vi "HV507 Write - Alt.vi"(8 "Error In":errorcluster, 10 "HV Data Bitmask":u64, 11 "LINX Resource":T1) -> (0 "Error Out":errorcluster, 3 "LINX Resource 2":T1)   [LabVIEW 2017]
doc: "Write 64-bit data to the 64 high voltage output channels of HV507.\n\nThis VI takes a 64 bit unigned integer as input and writes the bitwise data to HV507.\n\nArduino Microcontroller pins configured as follows:\nDIO 7 - ~BL\nDIO 8 - ~LE\nDIO 11 - DI\nDIO 13 - SCLK"
uses:
  <vilib>/MakerHub/LINX/Private/Type Defs/LINX Ref.ctl
  <vilib>/MakerHub/LINX/Private/Type Defs/Platform.ctl
  <vilib>/MakerHub/LINX/Private/Type Defs/Interface.ctl
  <vilib>/MakerHub/LINX/Private/Device/Type Defs/LINX Device Config.ctl
  <vilib>/MakerHub/LINX/Private/Device/Type Defs/TCP Config.ctl
  <vilib>/MakerHub/LINX/Private/Device/Type Defs/Channels.ctl
  <vilib>/MakerHub/LINX/Private/Type Defs/Peripherals/SPI/SPI Configuration.ctl
  <vilib>/MakerHub/LINX/Private/Type Defs/Peripherals/SPI/SPI Bit Order.ctl
  <vilib>/MakerHub/LINX/Private/Type Defs/Peripherals/SPI/SPI Mode.ctl
  <vilib>/MakerHub/LINX/Public/Peripherals/SPI/SPI CS Config.ctl
  <vilib>/MakerHub/LINX/Private/Type Defs/Peripherals/SPI/SPI CS Logic Level.ctl
  <vilib>/MakerHub/LINX/Public/Peripherals/SPI/SPI Write Read 1 Frame.vi
  <vilib>/MakerHub/LINX/Public/Peripherals/SPI/SPI Write Read N Frames.vi
  <vilib>/MakerHub/LINX/Private/Local IO/LinxSpiWriteRead.vi
  <vilib>/MakerHub/LINX/Public/Utilities/Check Channel.vi
  <vilib>/MakerHub/LINX/Private/Utilties/Generate Error.vi
  <vilib>/MakerHub/LINX/LMH-LINX.lvlib
  <vilib>/MakerHub/LINX/Private/Device/Device.lvlib
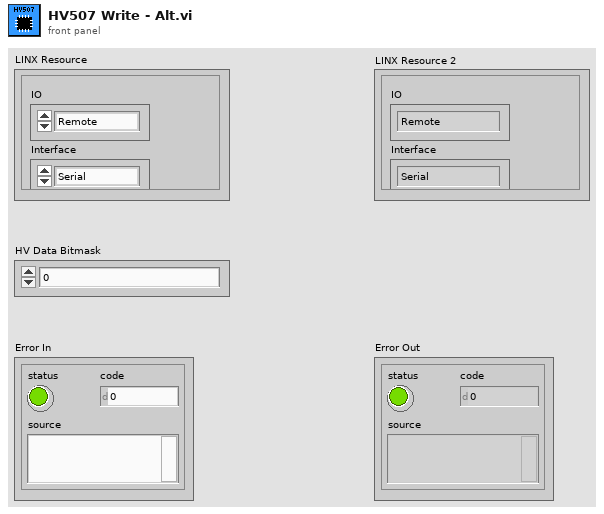
[diagram p1: front panel]
types:
  T1 = typedef "LMH-LINX.lvlib/LINX Ref.ctl" = cluster{"IO":T2, "Interface":T3, "LINX Device Config":T4}
  T2 = typedef "LMH-LINX.lvlib/Platform.ctl" = enum16{"Remote", "Local"}
  T3 = typedef "LMH-LINX.lvlib/Interface.ctl" = enum16{"Serial", "TCP"}
  T4 = typedef "LMH-LINX.lvlib/Device.lvlib/LINX Device Config.ctl" = cluster{"Interface":T3, "COM Port":refnum<visa-resource-name>, "TCP Configuration":T5, "Device Family":u8, "Device ID":u8, "Device Name":string, "TCP Ref":refnum<k5>, "Channels":T6}
  T5 = typedef "LMH-LINX.lvlib/Device.lvlib/TCP Config.ctl" = cluster{"IP Address":string, "Port":u16}
  T6 = typedef "LMH-LINX.lvlib/Channels.ctl" = cluster{"DI":u8[], "DO":u8[], "AI":u8[], "AO":u8[], "PWM":u8[], "QE":u8[], "UART":u8[], "I2C 2":u8[], "SPI":u8[], "CAN":u8[], "Servo":u8[], "AI Ref (V)":dbl, "AI Resolution (Bits)":u8, "AO Ref (V)":dbl, "AO Resolution (Bits)":u8}
  T7 = typedef "LMH-LINX.lvlib/SPI CS Config.ctl" = cluster{"CS Channel":u8, "CS Logic Level":T8}
  T8 = typedef "LMH-LINX.lvlib/SPI CS Logic Level.ctl" = enum8{"Active Low", "Active High"}
  T9 = typedef "LMH-LINX.lvlib/SPI Configuration.ctl" = cluster{"Clock Frequency":u32, "Bit Order":T10, "SPI Mode":T11}
  T10 = typedef "LMH-LINX.lvlib/SPI Bit Order.ctl" = enum8{"LSb First", "MSb First"}
  T11 = typedef "LMH-LINX.lvlib/SPI Mode.ctl" = enum8{"Mode 0", "Mode 1", "Mode 2", "Mode 3"}
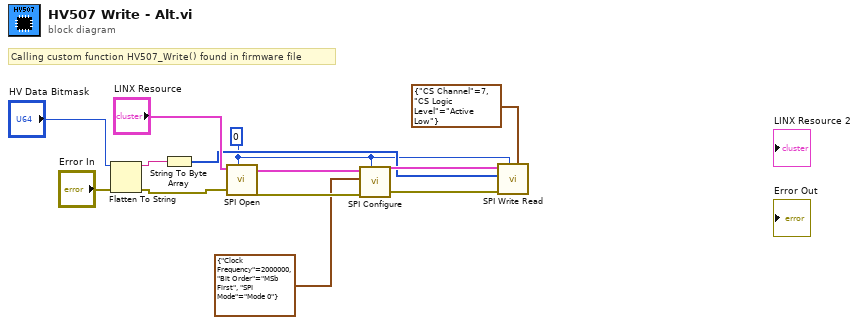
[diagram p0: block diagram]
diagram:
  w2 = u8 0 ("SPI Channel (0)")
  # "Calling custom function HV507_Write() found in firmware file"
  n1 = Flatten To String(anything="HV Data Bitmask", error in (no error)="Error In") -> (data string=w11:string, error out=w10:errorcluster)  [unwired: 2 in, 1 out]
  n2 = String To Byte Array(string=w11) -> (unsigned byte array=w3:u8[])
  n3 = call <vilib>:"SPI Open.vi"("SPI Channel (0)"=w2, "Error In"=w10, "LINX Resource"="LINX Resource") -> ("Error Out"=w8:errorcluster, "LINX Resource"=w7:T1)  [unwired: 7 in]
  n4 = call <vilib>:"SPI Configure.vi"("SPI Channel (0)"=w2, "Error In"=w8, "SPI Configuration"=T9 {"Clock Frequency"=2000000, "Bit Order"=enum."MSb First", "SPI Mode"=enum."Mode 0"}, "LINX Resource"=w7) -> ("Error Out"=w5:errorcluster, "LINX Resource"=w4:T1)  [unwired: 5 in, 1 out]
  n5 = call-poly <vilib>:"SPI Write Read.vi"("CS Configuration"=T7 {"CS Channel"=7, "CS Logic Level"=enum."Active Low"}, "SPI Channel (0)"=w2, "Error In"=w5, "Data"=w3, "LINX Resource"=w4) -> ()  [unwired: 4 in, 3 out]
